vi "Analysis Vol. 3 CSV Read.vi"() -> ()   [LabVIEW 2014] (continued)
        n138 = Bundle(w213, w212) -> (w214:cluster{dbl, dbl})  [unwired: 1 in]
        n139 = Delete From Array(array=w183, index (row)=0 ("disabled index (col)")) -> (array with subset deleted=w233:dbl[][])  [unwired: 2 in, 1 out]
        n140 = property on="Choose Range:" class="Slide (strict)"("Scale.Maximum"=w213, "Scale.Minimum"=w212, "Value"=w214) -> ()  [unwired: 2 in, 2 out]
        n141 = property on="Range 2" class="Slide (strict)"("Scale.Maximum"=w213) -> ()  [unwired: 2 in, 2 out]
        n142 = property on="Range 3" class="Slide (strict)"("Scale.Maximum"=w213) -> ()  [unwired: 2 in, 2 out]
        n143 = property on="Range 4" class="Slide (strict)"("Scale.Maximum"=w213) -> ()  [unwired: 2 in, 2 out]
        n144 = Reshape Array("Well Names", w227) -> (w224:string[])
        n145 = Reshape Array("Concetrations", w227) -> (w228:dbl[])
        n146 = local read "96-well"() -> (w241:bool[][])
        n147 = Reshape Array(w241, w221) -> (w219:bool[])
        n148 = Decrement(x=w221) -> (x-1=w222:i32)
        n149 = Reverse 1D Array(array=w219) -> (reversed array=w220:bool[])
        n150 = for {
          shift-right: [w274] -> w236
          shift-left: w234 -> [w269]
          shift-right: [w272] -> w237
          shift-left: w233 -> [w273]
          shift-right: [w270] -> w217
          shift-left: w218 -> [w271]
          tunnel: w220 -> [w268] mode=indexing
          tunnel: w222 -> [w265]
          shift-right: [w263] -> w225
          shift-left: w224 -> [w264]
          shift-right: [w261] -> w229
          shift-left: w228 -> [w262]
          i -> [w267]
          n151 = Subtract(x=w265, y=w267) -> (x-y=w266:i32)
          n152 = case shown="False" w268 {
            tunnel: w269 -> [w284 w290]
            tunnel: [w285 w290] -> w274
            tunnel: w273 -> [w283 w289]
            tunnel: [w282 w289] -> w272
            tunnel: w271 -> [w281 w288]
            tunnel: [w280 w288] -> w270
            tunnel: w266 -> [w276 _]
            tunnel: w264 -> [w279 w287]
            tunnel: [w278 w287] -> w263
            tunnel: [w275 w286] -> w261
            tunnel: w262 -> [w277 w286]
            frame False {
              n153 = Delete From Array(array=w284, index (row)=w276) -> (array with subset deleted=w285:dbl[][])  [unwired: 2 in, 1 out]
              n154 = Delete From Array(array=w283, index (row)=w276) -> (array with subset deleted=w282:dbl[][])  [unwired: 2 in, 1 out]
              n155 = Delete From Array(array=w281, index (row)=w276) -> (array with subset deleted=w280:dbl[][])  [unwired: 2 in, 1 out]
              n156 = Delete From Array(array=w279, index=w276) -> (array with subset deleted=w278:string[])  [unwired: 1 in, 1 out]
              n157 = Delete From Array(array=w277, index=w276) -> (array with subset deleted=w275:dbl[])  [unwired: 1 in, 1 out]
            }
            frame True {
            }
          }
        }
        "Well Names" <- w225
        "Concetrations" <- w229
        "Dye 1/Melting" <- w236
        "Dye 2" <- w237
        "reference" <- w217
        n158 = for {
          tunnel: w216 -> [w260]
          tunnel: w236 -> [w259] mode=indexing
          tunnel: w237 -> [w258] mode=indexing
          tunnel: [w257] -> w238 mode=indexing
          tunnel: [w256] -> w239 mode=indexing
          tunnel: [w255] -> w240 mode=indexing
          n159 = Bundle(w260, w259) -> (w257:cluster{dbl[], dbl[]})  [unwired: 1 in]
          n160 = Bundle(w260, w258) -> (w256:cluster{dbl[], dbl[]})  [unwired: 1 in]
          n161 = Bundle(w260, w259) -> (w255:cluster{dbl[], dbl[]})  [unwired: 1 in]
        }
        "Dye 2: G1" <- w239
        "Dye 1: G1" <- w238
        "Melting G1" <- w240
        n162 = for {
          tunnel: w217 -> [w254] mode=indexing
          tunnel: [w253] -> w215 mode=indexing
          tunnel: w216 -> [w252]
          n163 = Bundle(w252, w254) -> (w253:cluster{dbl[], dbl[]})  [unwired: 1 in]
        }
        "REFERENCE G" <- w215
      }
      event "Range 2": Value Change {
        n164 = event-data() -> ()  [unwired: 1 in, 1 out]
        n165 = Unbundle("Range 2") -> (w294:dbl, w293:dbl)
        n166 = Max & Min(x=w294, y=w293) -> (max(x,y)=w292:dbl, min(x,y)=w291:dbl)
        n167 = property on="Dye1: G2" class="XYGraph (strict)"("XScale.Maximum"=w292, "XScale.Minimum"=w291) -> ()  [unwired: 2 in, 2 out]
      }
      event "Range 3": Value Change {
        n168 = event-data() -> ()  [unwired: 1 in, 1 out]
        n169 = Unbundle("Range 3") -> (w296:dbl, w297:dbl)
        n170 = Max & Min(x=w296, y=w297) -> (max(x,y)=w298:dbl, min(x,y)=w299:dbl)
        n171 = property on="Dye 5" class="XYGraph (strict)"("XScale.Maximum"=w298, "XScale.Minimum"=w299) -> ()  [unwired: 2 in, 2 out]
      }
      event "Range 4": Value Change {
        n172 = event-data() -> ()  [unwired: 1 in, 1 out]
        n173 = Unbundle("Range 4") -> (w301:dbl, w302:dbl)
        n174 = Max & Min(x=w301, y=w302) -> (max(x,y)=w304:dbl, min(x,y)=w305:dbl)
        n175 = property on="Dye1: G4" class="XYGraph (strict)"("XScale.Maximum"=w304, "XScale.Minimum"=w305) -> ()  [unwired: 2 in, 2 out]
      }
      event "Melting G1", "Melting G2", "Melting: G3": Cursor Move; "Intercalating/\nQuenching", "T[°C]", "conc [nM]": Value Change {
        w350 = 0.0019872041  # R
        w361 = 273.15
        # "lower T [°C]"
        # "points between\ncursors in G3"
        # "Jean-Louis Mergny and Laurent Lacroix. \nOligonucleotides. December 2003,\n13(6): 515-537. \ndoi:10.1089/154545703322860825."
        # "cursor pair green"
        # "cursor pair yellow"
        # "Fit baselines with cursors and make a bound fraction\nplot out of the meltcurve"
        # "stepsize"
        n176 = event-data() -> ()  [unwired: 1 in, 1 out]
        n177 = local read "Temp/Time\nranged"() -> (w324:dbl[])
        n178 = local read "Dye1/Melting ranged"() -> (w329:dbl[][])
        n179 = property on="Melting G1" class="XYGraph (strict)"("Active Cursor"=u32 0, "Active Cursor"=u32 1) -> ("Cursor.Cursor X"=w385:dbl, "Cursor.Cursor X"=w384:dbl)  [unwired: 2 in, 2 out]
        n180 = property on="Melting G3" class="XYGraph (strict)"("Active Cursor"=u32 1, "Active Cursor"=u32 0) -> ("Cursor.Cursor X"=w365:dbl, "Cursor.Cursor X"=w364:dbl)  [unwired: 2 in, 2 out]
        n181 = property on="Melting G1" class="XYGraph (strict)"("Active Cursor"=u32 2, "Active Cursor"=u32 3) -> ("Cursor.Cursor X"=w376:dbl, "Cursor.Cursor X"=w375:dbl)  [unwired: 2 in, 2 out]
        n182 = Index Array(array=w324, index=1) -> (element=w381:dbl)
        n183 = Index Array(array=w324, index=0) -> (element=w380:dbl)
        n184 = Subtract(x=w381, y=w380) -> ()  [unwired: 1 out]
        n185 = Reciprocal(x=w365) -> (1/x=w363:dbl)
        n186 = Reciprocal(x=w364) -> (1/x=w362:dbl)
        n187 = Max & Min(x=w385, y=w384) -> (max(x,y)=w336:dbl, min(x,y)=w335:dbl)
        n188 = Max & Min(x=w376, y=w375) -> (max(x,y)=w342:dbl, min(x,y)=w343:dbl)
        n189 = Subtract(x=w363, y=w361) -> (x-y=w359:dbl)
        n190 = Subtract(x=w362, y=w361) -> (x-y=w360:dbl)
        n191 = Max & Min(x=w359, y=w360) -> (max(x,y)=w325:dbl, min(x,y)=w316:dbl)
        "Upper T [°C]" <- w325
        "Lower T [°C]" <- w316
        n192 = Threshold 1D Array(2:w343, 3:w324) -> (0:w340:dbl)  [unwired: 1 in]
        n193 = Threshold 1D Array(2:w342, 3:w324) -> (0:w341:dbl)  [unwired: 1 in]
        n194 = Threshold 1D Array(2:w335, 3:w324) -> (0:w333:dbl)  [unwired: 1 in]
        n195 = Threshold 1D Array(2:w336, 3:w324) -> (0:w334:dbl)  [unwired: 1 in]
        n196 = Round Toward +Infinity(x=w341) -> (ceil(x): smallest int >= x=w338:dbl)
        n197 = Round Toward -Infinity(1:w340) -> (0:w337:dbl)
        n198 = Round Toward +Infinity(x=w334) -> (ceil(x): smallest int >= x=w332:dbl)
        n199 = Round Toward -Infinity(1:w333) -> (0:w331:dbl)
        n200 = Threshold 1D Array(2:w316, 3:w324) -> (0:w322:dbl)  [unwired: 1 in]
        n201 = Threshold 1D Array(2:w325, 3:w324) -> (0:w323:dbl)  [unwired: 1 in]
        n202 = Subtract(x=w338, y=w337) -> (x-y=w339:dbl)
        n203 = Subtract(x=w332, y=w331) -> (x-y=w327:dbl)
        n204 = Increment(x=w327) -> (x+1=w326:dbl)
        n205 = Round Toward +Infinity(x=w323) -> (ceil(x): smallest int >= x=w321:dbl)
        n206 = Round Toward -Infinity(1:w322) -> (0:w318:dbl)
        n207 = Increment(x=w339) -> (x+1=w328:dbl)
        n208 = property on="Melting G2" class="XYGraph (strict)"("Active Cursor"=u32 0, "Active Cursor"=u32 1) -> ("Cursor.Cursor X"=w371:dbl, "Cursor.Cursor Y"=w310:dbl, "Cursor.Cursor X"=w370:dbl, "Cursor.Cursor Y"=w309:dbl)  [unwired: 2 in, 2 out]
        n209 = Subtract(x=w321, y=w318) -> (x-y=w320:dbl)
        n210 = Increment(x=w320) -> (x+1=w319:dbl)
        n211 = Array Subset(array=w329, index (col)=w331, length (col)=w326) -> (w387:dbl[][])  [unwired: 2 in]
        "Baseline1" <- w387
        n212 = Array Subset(array=w324, index=w331, length=w326) -> (w386:dbl[])
        "Baseline1T" <- w386
        n213 = Array Subset(array=w329, index (col)=w337, length (col)=w328) -> (w374:dbl[][])  [unwired: 2 in]
        "Baseline2" <- w374
        n214 = Array Subset(array=w324, index=w337, length=w328) -> (w373:dbl[])
        "Baseline2T" <- w373
        n215 = Max & Min(x=w310, y=w309) -> (max(x,y)=→"Upper fraction":dbl, min(x,y)=→"Lower fraction":dbl)
        n216 = local read "Dye 1: G1"() -> (w379:cluster{"Y":dbl[], "Y":dbl[]}[])
        n217 = for {
          tunnel: w387 -> [w453] mode=indexing
          tunnel: w386 -> [w450]
          shift-right: [w452] -> w330
          shift-left: w379 -> [w407]
          tunnel: w329 -> [w437] mode=indexing
          tunnel: w374 -> [w449] mode=indexing
          tunnel: w373 -> [w447]
          tunnel: w324 -> [w398]
          tunnel: w343 -> [w441]
          tunnel: w335 -> [w440]
          tunnel: [w439] -> w372 mode=indexing
          tunnel: w371 -> [w435]
          tunnel: w370 -> [w434]
          tunnel: w316 -> [w394]
          tunnel: w319 -> [w423]
          tunnel: [w415] -> w367 mode=indexing
          tunnel: [w413] -> w352 mode=indexing
          tunnel: [w412] -> w353 mode=indexing
          tunnel: [w410] -> w358 mode=indexing
          tunnel: [w409] -> w357 mode=indexing
          tunnel: [w408] -> w356 mode=indexing
          tunnel: [w396] -> w317 mode=indexing
          w419 = 0.0019872041  # R
          w430 = 1e-09 ("x")
          # "lower T [°C]"
          # "ln(Ka) between cursors in G3"
          # "1/Temp between cursors in G3"
          # "Graph 3"
          # "fraction \nbound"
          # "index of lower T in G3"
          # "points between\ncursors in G3"
          # "Temp between cursors in G2"
          # "Fraction=(Higher Baseline - Signal)\n/(Higher Baseline - Lower Baseline)"
          # "green baseline"
          # "yellow baseline"
          # "which baseline is upper?"
          # "meltcurve"
          n218 = local read "Intercalating/\nQuenching"() -> (w436:bool)
          n219 = Max & Min(x=w435, y=w434) -> (max(x,y)=w391:dbl, min(x,y)=w390:dbl)
          n220 = call <vilib>:"Linear Fit.vi"("Y"=w453, "X"=w450) -> ("Best Linear Fit"=w451:dbl[], "slope"=w442:dbl, "intercept"=w443:dbl)  [unwired: 9 in, 2 out]
          n221 = call <vilib>:"Linear Fit.vi"("Y"=w449, "X"=w447) -> ("Best Linear Fit"=w448:dbl[], "slope"=w444:dbl, "intercept"=w445:dbl)  [unwired: 9 in, 2 out]
          n222 = for {
            tunnel: w443 -> [w473]
            tunnel: w442 -> [w476]
            tunnel: [w474] -> w401 mode=indexing
            tunnel: w398 -> [w472] mode=indexing
            n223 = Multiply(x=w476, y=w472) -> (x*y=w475:dbl)
            n224 = Add(x=w473, y=w475) -> (x+y=w474:dbl)
          }
          n225 = case shown="False" w436 {
            tunnel: [w454 w459] -> w400
            tunnel: w441 -> [w456 w458]
            tunnel: w440 -> [w455 w457]
            frame False {
              n226 = Greater?(x=w456, y=w455) -> (0:w454:bool)
            }
            frame True {
              n227 = Less?(x=w458, y=w457) -> (x < y?=w459:bool)
            }
          }
          n228 = for {
            tunnel: w445 -> [w477]
            tunnel: w444 -> [w479]
            tunnel: [w481] -> w438 mode=indexing
            tunnel: w398 -> [w480] mode=indexing
            # "stretch the fit over the \nwhole x-axis"
            n229 = Multiply(x=w480, y=w479) -> (x*y=w478:dbl)
            n230 = Add(x=w478, y=w477) -> (x+y=w481:dbl)
          }
          n231 = Bundle(w450, "Best Linear Fit"=w451) -> (w399:cluster{dbl[], "Best Linear Fit":dbl[]})  [unwired: 1 in]
          n232 = Bundle(w447, "Best Linear Fit"=w448) -> (w446:cluster{dbl[], "Best Linear Fit":dbl[]})  [unwired: 1 in]
          n233 = Threshold 1D Array(2:w390, 3:w398) -> (0:w405:dbl)  [unwired: 1 in]
          n234 = Threshold 1D Array(2:w391, 3:w398) -> (0:w406:dbl)  [unwired: 1 in]
          n235 = Insert Into Array(array=w407, new element #1=w446, new element #2=w399) -> (w452:cluster{"Y":dbl[], "Y":dbl[]}[])  [unwired: 1 in]
          n236 = Round Toward +Infinity(x=w406) -> (ceil(x): smallest int >= x=w404:dbl)
          n237 = Round Toward -Infinity(1:w405) -> (0:w403:dbl)
          n238 = Subtract(x=w404, y=w403) -> (x-y=w402:dbl)
          n239 = Increment(x=w402) -> (x+1=w397:dbl)
          n240 = Array Subset(array=w398, index=w403, length=w397) -> (w395:dbl[])
          n241 = case shown="False" w400 {
            tunnel: w437 -> [w462 w468]
            tunnel: w401 -> [w460 w467]
            tunnel: w438 -> [w461 w466]
            tunnel: [w463 w469] -> w410
            frame False {
              n242 = Subtract(x=w461, y=w460) -> (x-y=w464:dbl[])
              n243 = Subtract(x=w461, y=w462) -> (x-y=w465:dbl[])
              n244 = Divide(x=w465, y=w464) -> (x/y=w463:dbl[])
            }
            frame True {
              n245 = Subtract(x=w467, y=w468) -> (x-y=w471:dbl[])
              n246 = Subtract(x=w467, y=w466) -> (x-y=w470:dbl[])
              n247 = Divide(x=w471, y=w470) -> (x/y=w469:dbl[])
            }
          }
          n248 = Threshold 1D Array(2:w394, 3:w395) -> (0:w393:dbl)  [unwired: 1 in]
          n249 = Add(x=w395, y=273.15) -> (x+y=w433:dbl[])
          n250 = Reciprocal(x=w433) -> (1/x=w422:dbl[])
          "1/K" <- w422
          n251 = Round Toward -Infinity(1:w393) -> (0:w392:dbl)
          n252 = Array Subset(array=w410, index=w403, length=w397) -> (w411:dbl[])
          n253 = Bundle("Temp/Time\nranged"=w398, w410) -> (w439:cluster{"Temp/Time\nranged":dbl[], dbl[]})  [unwired: 1 in]
          n254 = Subtract(x=w411, y=1) -> (x-y=w431:dbl[])
          n255 = Compound Arithmetic op=MULTIPLY(w431, w430, "conc [nM]") -> (w428:dbl[])
          n256 = Compound Arithmetic op=MULTIPLY(w411, w430, "conc [nM]") -> (w425:dbl[])
          n257 = Square(x=w428) -> (x^2=w427:dbl[])
          n258 = Reciprocal(x=w427) -> (1/x=w426:dbl[])
          n259 = Multiply(x=w426, y=w425) -> (x*y=w424:dbl[])
          n260 = Natural Logarithm(1:w424) -> (0:w409:dbl[])
          n261 = Bundle(w422, w409) -> (w415:cluster{dbl[], dbl[]})  [unwired: 1 in]
          n262 = Array Subset(array=w409, index=w392, length=w423) -> (w417:dbl[])
          n263 = Array Subset(array=w422, index=w392, length=w423) -> (w416:dbl[])
          "ArrhFitT" <- w416
          n264 = call <vilib>:"Linear Fit.vi"("Y"=w417, "X"=w416) -> ("Best Linear Fit"=w408:dbl[], "slope"=w418:dbl, "intercept"=w421:dbl)  [unwired: 9 in, 2 out]
          n265 = Bundle(w416, "Best Linear Fit"=w408) -> (w396:cluster{dbl[], "Best Linear Fit":dbl[]})  [unwired: 1 in]
          n266 = Multiply(x=w419, y=w418) -> (x*y=w414:dbl)
          n267 = Multiply(x=w421, y=w419) -> (x*y=w412:dbl)
          n268 = Negate(x=w414) -> (-x=w413:dbl)
        }
        "Melting G2" <- w372
        "deltaH\n[kcal/mol]" <- w352
        "deltaS \n[kcal/K*mol]" <- w353
        "Bound Fraction" <- w358
        "ArrhLn" <- w357
        "ArrhFit" <- w356
        n269 = Insert Into Array(array=w367, new element=w317) -> (→"Melting: G3":cluster{dbl[], dbl[]}[])  [unwired: 1 in]
        n270 = local write "Melting G1"(w330) -> ()
        n271 = Add(x="T[°C]", y=273.15) -> (x+y=w307:dbl)
        n272 = Multiply(x=w353, y=w307) -> (x*y=w351:dbl[])
        n273 = Subtract(x=w352, y=w351) -> (x-y=w308:dbl[])
        "deltaG(T)\n[kcal/mol]" <- w308
        n274 = Multiply(x=w307, y=w350) -> (x*y=w306:dbl)
        n275 = Divide(x=w308, y=w306) -> (x/y=w349:dbl[])
        n276 = Exponential(1:w349) -> (0:w348:dbl[])
        n277 = Multiply(x=1000000000, y=w348) -> (x*y=w314:dbl[])
        "Kd\n[nM]" <- w314
        n278 = Multiply(x=w314, y="kon [1/(s*nM)]") -> (x*y=→"koff \n[1/s]":dbl[])
        n279 = Reciprocal(x=w314) -> (1/x=→"Ka\n[1/nM]":dbl[])
      }
      event "To Igor Meltcurve": Value Change {
        n280 = event-data() -> ()  [unwired: 1 in, 6 out]
        n281 = case shown="True" "Melting Curves" {
          frame False {
          }
          frame True {
            n282 = local read "Dye1/Melting ranged"() -> (w547:dbl[][])
            n283 = local read "Dye 1/Melting"() -> (w539:dbl[][])
            n284 = local read "Well Names"() -> (w540:string[])
            n285 = local read "Baseline2"() -> (w541:dbl[][])
            n286 = local read "Baseline1"() -> (w542:dbl[][])
            n287 = local read "Temp/Time\nranged"() -> (w548:dbl[])
            n288 = local read "Temp/Time"() -> (w537:dbl[])
            n289 = local read "Baseline1T"() -> (w543:dbl[])
            n290 = local read "Baseline2T"() -> (w544:dbl[])
            n291 = for {
              tunnel: w540 -> [w551] mode=indexing
              tunnel: w539 -> [w550] mode=indexing
              n292 = Concatenate Strings("Melt_raw_" ("string"), w551) -> (w553:string)
              n293 = call "1D_Data_to_Igor.vi"("Wave Name"=w553, "Data"=w550) -> ()  [unwired: 9 in, 1 out]
            }
            n294 = for {
              tunnel: w540 -> [w563] mode=indexing
              tunnel: w547 -> [w562] mode=indexing
              n295 = Concatenate Strings("Melt_cut_" ("string"), w563) -> (w565:string)
              n296 = call "1D_Data_to_Igor.vi"("Wave Name"=w565, "Data"=w562) -> ()  [unwired: 9 in, 1 out]
            }
            n297 = for {
              tunnel: w540 -> [w559] mode=indexing
              tunnel: w541 -> [w558] mode=indexing
              n298 = Concatenate Strings("Melt_BL2_" ("string"), w559) -> (w561:string)
              n299 = call "1D_Data_to_Igor.vi"("Wave Name"=w561, "Data"=w558) -> ()  [unwired: 9 in, 1 out]
            }
            n300 = for {
              tunnel: w540 -> [w555] mode=indexing
              tunnel: w542 -> [w554] mode=indexing
              n301 = Concatenate Strings("Melt_BL1_" ("string"), w555) -> (w557:string)
              n302 = call "1D_Data_to_Igor.vi"("Wave Name"=w557, "Data"=w554) -> ()  [unwired: 9 in, 1 out]
            }
            n303 = call "1D_Data_to_Igor.vi"("Wave Name"="Melt_cut_Temperature" ("string"), "Data"=w548) -> ()  [unwired: 9 in, 1 out]
            n304 = call "1D_Data_to_Igor.vi"("Wave Name"="Melt_TemperatureBL1" ("string"), "Data"=w543) -> ()  [unwired: 9 in, 1 out]
            n305 = call "1D_Data_to_Igor.vi"("Wave Name"="Melt_TemperatureBL2" ("string"), "Data"=w544) -> ()  [unwired: 9 in, 1 out]
            n306 = call "1D_Data_to_Igor.vi"("Wave Name"="Melt_raw_Temperature" ("string"), "Data"=w537) -> ()  [unwired: 9 in, 1 out]
          }
        }
        n307 = case shown="True" "Bound Fraction" {
          frame False {
          }
          frame True {
            n308 = local read "Bound Fraction"() -> (w530:dbl[][])
            n309 = local read "Temp/Time\nranged"() -> (w529:dbl[])
            n310 = local read "Well Names"() -> (w531:string[])
            n311 = for {
              tunnel: w531 -> [w534] mode=indexing
              tunnel: w530 -> [w533] mode=indexing
              n312 = Concatenate Strings("Fraction_" ("string"), w534) -> (w536:string)
              n313 = call "1D_Data_to_Igor.vi"("Wave Name"=w536, "Data"=w533) -> ()  [unwired: 9 in, 1 out]
            }
            n314 = call "1D_Data_to_Igor.vi"("Wave Name"="Fraction_Temperature" ("string"), "Data"=w529) -> ()  [unwired: 9 in, 1 out]
          }
        }
        n315 = case shown="True" "Arrhenius Plot" {
          frame False {
          }
          frame True {
            n316 = local read "Well Names"() -> (w520:string[])
            n317 = local read "ArrhFit"() -> (w515:dbl[][])
            n318 = local read "ArrhLn"() -> (w518:dbl[][])
            n319 = for {
              tunnel: w520 -> [w522] mode=indexing
              tunnel: w518 -> [w526] mode=indexing
              tunnel: w515 -> [w524] mode=indexing
              n320 = Concatenate Strings("ArrhFit_" ("string"), w522) -> (w525:string)
              n321 = Concatenate Strings("Arrh_" ("string"), w522) -> (w528:string)
              n322 = call "1D_Data_to_Igor.vi"("Wave Name"=w525, "Data"=w524) -> ()  [unwired: 9 in, 1 out]
              n323 = call "1D_Data_to_Igor.vi"("Wave Name"=w528, "Data"=w526) -> ()  [unwired: 9 in, 1 out]
            }
            n324 = local read "ArrhFitT"() -> (w516:dbl[])
            n325 = local read "1/K"() -> (w519:dbl[])
            n326 = call "1D_Data_to_Igor.vi"("Wave Name"="Arrh_invT" ("string"), "Data"=w519) -> ()  [unwired: 9 in, 1 out]
            n327 = call "1D_Data_to_Igor.vi"("Wave Name"="ArrhFit_invT" ("string"), "Data"=w516) -> ()  [unwired: 9 in, 1 out]
          }
        }
        n328 = case shown="True" "Energies & Kd, Ka" {
          frame False {
          }
          frame True {
            w490 = "_" ("string")
            n329 = local read "kon [1/(s*nM)]"() -> (w488:dbl)
            n330 = local read "conc [nM]"() -> (w497:dbl)
            n331 = local read "deltaS \n[kcal/K*mol]"() -> (w514:dbl[])
            n332 = local read "T[°C]"() -> (w507:dbl)
            n333 = local read "deltaH\n[kcal/mol]"() -> (w510:dbl[])
            n334 = local read "Well Names"() -> (w500:string[])
            n335 = Number To Decimal String(number=w507) -> (decimal integer string=w499:string)  [unwired: 1 in]
            n336 = Number To Decimal String(number=w497) -> (decimal integer string=w491:string)  [unwired: 1 in]
            n337 = Number To Fractional String(number=w488, width (-)=5, precision (6)=4) -> (F-format string=w489:string)  [unwired: 1 in]
            n338 = call "1D_Strings_to_Igor_with_Prefix.vi"("Wave Name"="Samples" ("string"), "Data"=w500) -> ()  [unwired: 9 in, 1 out]
            n339 = call "1D_Data_to_Igor.vi"("Wave Name"="deltaS_kcal_K_mol" ("string"), "Data"=w514) -> ()  [unwired: 9 in, 1 out]
            n340 = call "1D_Data_to_Igor.vi"("Wave Name"="deltaH_kcal_mol" ("string"), "Data"=w510) -> ()  [unwired: 9 in, 1 out]
            n341 = local read "deltaG(T)\n[kcal/mol]"() -> (w511:dbl[])
            n342 = Concatenate Strings("deltaG_kcal_mol_" ("string"), w499) -> (w502:string)
            n343 = Concatenate Strings("koff_" ("string"), w499, w490, w491, w490, w489) -> (w493:string)
            n344 = local read "koff \n[1/s]"() -> (w498:dbl[])
            n345 = call "1D_Data_to_Igor.vi"("Wave Name"=w502, "Data"=w511) -> ()  [unwired: 9 in, 1 out]
            n346 = call "1D_Data_to_Igor.vi"("Wave Name"=w493, "Data"=w498) -> ()  [unwired: 9 in, 1 out]
            n347 = Concatenate Strings("Kd_nM_" ("string"), w499, "_" ("string"), w491) -> (w495:string)
            n348 = Concatenate Strings("Ka_nM_" ("string"), w499, "_" ("string"), w491) -> (w505:string)
            n349 = local read "Kd\n[nM]"() -> (w508:dbl[])
            n350 = local read "Ka\n[1/nM]"() -> (w509:dbl[])
            n351 = call "1D_Data_to_Igor.vi"("Wave Name"=w495, "Data"=w508) -> ()  [unwired: 9 in, 1 out]
            n352 = call "1D_Data_to_Igor.vi"("Wave Name"=w505, "Data"=w509) -> ()  [unwired: 9 in, 1 out]
          }
        }
      }
      event "Row": Value Change {
        n353 = event-data() -> ("NewVal"=w581:bool[], "OldVal"=w580:bool[])  [unwired: 1 in]
        n354 = Boolean To (0,1)(Boolean=w581) -> (0, 1=w579:i16[])
        n355 = Boolean To (0,1)(Boolean=w580) -> (0, 1=w578:i16[])
        n356 = Subtract(x=w579, y=w578) -> (x-y=w577:i16[])
        n357 = Absolute Value(x=w577) -> (abs(x)=w576:i16[])
        n358 = Array Max & Min(array=w576) -> (max index (indices)=w569:i32)  [unwired: 3 out]
        n359 = Index Array(array="96-well", index (row)=w569) -> (element=w570:bool[])  [unwired: 1 in]
        n360 = Boolean To (0,1)(Boolean=w570) -> (0, 1=w571:i16[])
        n361 = Multiply Array Elements(1:w571) -> (0:w572:i16)
        n362 = Equal To 0?(x=w572) -> (x = 0?=w573:bool)
        n363 = Select(t=bool[] [TRUE, TRUE, TRUE, TRUE, TRUE, TRUE, TRUE, TRUE, TRUE, TRUE, TRUE, TRUE] ("new element/subarray"), s=w573, f=bool[] [FALSE, FALSE, FALSE, FALSE, FALSE, FALSE, FALSE, FALSE, FALSE, FALSE, FALSE, FALSE] ("new element/subarray")) -> (s? t:f=w574:bool[])
        n364 = Replace Array Subset(array="96-well", new element=w574, index (row)=w569) -> (w575:bool[][])  [unwired: 1 in]
        n365 = local write "96-well"(w575) -> ()
      }
      event "All": Value Change {
        n366 = event-data() -> ()  [unwired: 1 in, 1 out]
        n367 = local read "96-well"() -> (w582:bool[][])
        n368 = Boolean To (0,1)(Boolean=w582) -> (0, 1=w588:i16[][])
        n369 = Multiply Array Elements(1:w588) -> (0:w586:i16)
        n370 = Equal To 0?(x=w586) -> (x = 0?=w585:bool)
        n371 = Select(t=bool[][] [[TRUE, TRUE, TRUE, TRUE, TRUE, TRUE, TRUE, TRUE, TRUE, TRUE, TRUE, TRUE], [TRUE, TRUE, TRUE, TRUE, TRUE, TRUE, TRUE, TRUE, TRUE, TRUE, TRUE, TRUE], [TRUE, TRUE, TRUE, TRUE, TRUE, TRUE, TRUE, TRUE, TRUE, TRUE, TRUE, TRUE], [TRUE, TRUE, TRUE, TRUE, TRUE, TRUE, TRUE, TRUE, TRUE, TRUE, TRUE, TRUE], [TRUE, TRUE, TRUE, TRUE, TRUE, TRUE, TRUE, TRUE, TRUE, TRUE, TRUE, TRUE], [TRUE, TRUE, TRUE, TRUE, TRUE, TRUE, TRUE, TRUE, TRUE, TRUE, TRUE, TRUE], [TRUE, TRUE, TRUE, TRUE, TRUE, TRUE, TRUE, TRUE, TRUE, TRUE, TRUE, TRUE], [TRUE, TRUE, TRUE, TRUE, TRUE, TRUE, TRUE, TRUE, TRUE, TRUE, TRUE, TRUE]] ("96-well 2"), s=w585, f=bool[][] [[FALSE, FALSE, FALSE, FALSE, FALSE, FALSE, FALSE, FALSE, FALSE, FALSE, FALSE, FALSE], [FALSE, FALSE, FALSE, FALSE, FALSE, FALSE, FALSE, FALSE, FALSE, FALSE, FALSE, FALSE], [FALSE, FALSE, FALSE, FALSE, FALSE, FALSE, FALSE, FALSE, FALSE, FALSE, FALSE, FALSE], [FALSE, FALSE, FALSE, FALSE, FALSE, FALSE, FALSE, FALSE, FALSE, FALSE, FALSE, FALSE], [FALSE, FALSE, FALSE, FALSE, FALSE, FALSE, FALSE, FALSE, FALSE, FALSE, FALSE, FALSE], [FALSE, FALSE, FALSE, FALSE, FALSE, FALSE, FALSE, FALSE, FALSE, FALSE, FALSE, FALSE], [FALSE, FALSE, FALSE, FALSE, FALSE, FALSE, FALSE, FALSE, FALSE, FALSE, FALSE, FALSE], [FALSE, FALSE, FALSE, FALSE, FALSE, FALSE, FALSE, FALSE, FALSE, FALSE, FALSE, FALSE]] ("96-well 2")) -> (s? t:f=w587:bool[][])
        n372 = local write "96-well"(w587) -> ()
      }
      event "Line": Value Change {
        n373 = event-data() -> ("NewVal"=w604:bool[], "OldVal"=w603:bool[])  [unwired: 1 in]
        n374 = Boolean To (0,1)(Boolean=w604) -> (0, 1=w602:i16[])
        n375 = Boolean To (0,1)(Boolean=w603) -> (0, 1=w601:i16[])
        n376 = Subtract(x=w602, y=w601) -> (x-y=w600:i16[])
        n377 = Absolute Value(x=w600) -> (abs(x)=w599:i16[])
        n378 = local read "96-well"() -> (w589:bool[][])
        n379 = Array Max & Min(array=w599) -> (max index (indices)=w592:i32)  [unwired: 3 out]
        n380 = Index Array(array=w589, index (col)=w592) -> (element=w593:bool[])  [unwired: 1 in]
        n381 = Boolean To (0,1)(Boolean=w593) -> (0, 1=w594:i16[])
        n382 = Multiply Array Elements(1:w594) -> (0:w595:i16)
        n383 = Equal To 0?(x=w595) -> (x = 0?=w596:bool)
        n384 = Select(t=bool[] [TRUE, TRUE, TRUE, TRUE, TRUE, TRUE, TRUE, TRUE] ("Row 2"), s=w596, f=bool[] [FALSE, FALSE, FALSE, FALSE, FALSE, FALSE, FALSE, FALSE] ("Row 3")) -> (s? t:f=w597:bool[])
        n385 = Replace Array Subset(array=w589, new element=w597, index (col)=w592) -> (w598:bool[][])  [unwired: 1 in]
        n386 = local write "96-well"(w598) -> ()
      }
      event "96-well": Value Change {
        n387 = event-data() -> ()  [unwired: 1 in, 2 out]
        n388 = local read "Reference \non/off"() -> (w605:bool)
        n389 = property on="Reference \non/off" class="Bool (strict)"("Val(Sgnl)"=w605) -> ()  [unwired: 2 in, 2 out]
        n390 = local read "Load Dye 2"() -> (w606:path)
        n391 = property on="Load Dye 2" class="Path"("Val(Sgnl)"=w606) -> ()  [unwired: 2 in, 2 out]
      }
      event "Dye 1: G1": Cursor Move; "Update Dye1: G2": Value Change {
        # "Dye1array"
        n392 = event-data() -> ()  [unwired: 1 in, 1 out]
        n393 = local read "Dye1/Melting ranged"() -> (w607:dbl[][])
        n394 = case shown="True" "I - I0" {
          tunnel: w607 -> [w645 w647]
          tunnel: [w645 w646] -> w617
          frame False {
          }
          frame True {
            # "Subtrac I0"
            n395 = for {
              tunnel: w647 -> [w649] mode=indexing
              tunnel: [w648] -> w646 mode=indexing
              n396 = Index Array(array=w649, index=0) -> (element=w650:dbl)
              n397 = Subtract(x=w649, y=w650) -> (x-y=w648:dbl[])
            }
          }
        }
        n398 = local read "Temp/Time\nranged"() -> (w608:dbl[])
        n399 = case shown="True" "Baseline Correction" {
          tunnel: w617 -> [w656 w688]
          tunnel: w608 -> [w658 w681]
          tunnel: "Concentrations" -> [_ w685]
          tunnel: "Invert" -> [w655 w683]
          tunnel: [w656 w680] -> w615
          tunnel: [w657 w682] -> w614
          tunnel: "Normalize" -> [w653 w678]
          frame False {
            n400 = case shown="False" w655 {
              tunnel: [w667 w674] -> w654
              tunnel: w656 -> [w668 w674]
              frame True {
                n401 = for {
                  tunnel: w668 -> [w670] mode=indexing
                  tunnel: [w669] -> w667 mode=indexing
                  n402 = Array Max & Min(array=w670) -> (max value=w671:dbl)  [unwired: 3 out]
                  n403 = Multiply(x=w670, y=-1.0) -> (x*y=w672:dbl[])
                  n404 = Add(x=w672, y=w671) -> (x+y=w669:dbl[])
                }
              }
              frame False {
              }
            }
            n405 = case shown="True" w653 {
              tunnel: [w659 w660] -> w652
              tunnel: w654 -> [w659 w661]
              frame False {
              }
              frame True {
                n406 = for {
                  tunnel: w661 -> [w665] mode=indexing
                  tunnel: [w662] -> w660 mode=indexing
                  n407 = Array Max & Min(array=w665) -> (min value=w666:dbl)  [unwired: 3 out]
                  n408 = Subtract(x=w665, y=w666) -> (x-y=w663:dbl[])
                  n409 = Array Max & Min(array=w663) -> (max value=w664:dbl)  [unwired: 3 out]
                  n410 = Divide(x=w663, y=w664) -> (x/y=w662:dbl[])
                }
              }
            }
            n411 = local write "Dye1withBaselineCorrection"(w652) -> ()
            n412 = for {
              tunnel: [w677] -> w657 mode=indexing
              tunnel: w658 -> [w676]
              tunnel: w652 -> [w675] mode=indexing
              # "Create Plots"
              n413 = Bundle("Temp/Time\nranged"=w676, "Dye1/Melting ranged"=w675) -> (w677:T4)  [unwired: 1 in]
            }
            n414 = local write "Dye1: G2"(w657) -> ()
          }
          frame True {
            # "I-I0"
            n415 = property on="Dye 1: G1" class="XYGraph (strict)"("Active Cursor"=u32 0, "Active Cursor"=u32 1) -> ("Cursor.Cursor X"=w699:dbl, "Cursor.Cursor X"=w700:dbl)  [unwired: 2 in, 2 out]
            n416 = Array Size(array=w688) -> (size(s)=w691:i32[])
            n417 = Index Array(array=w691, index=1) -> (element=w689:i32)
            n418 = Max & Min(x=w699, y=w700) -> (max(x,y)=w695:dbl, min(x,y)=w692:dbl)
            n419 = Subtract(x=w695, y=w692) -> (x-y=w693:dbl)
            n420 = Array Subset(array=w688, index (col)=w692, length (col)=w693) -> (w694:dbl[][])  [unwired: 2 in]
            n421 = Array Subset(array=w681, index=w692, length=w693) -> (w696:dbl[])
            n422 = for {
              tunnel: w694 -> [w752] mode=indexing
              tunnel: w696 -> [w751]
              tunnel: w689 -> [w750]
              tunnel: [w745] -> w687 mode=indexing
              n423 = call <vilib>:"Linear Fit.vi"("Y"=w752, "X"=w751) -> ("slope"=w746:dbl, "intercept"=w747:dbl)  [unwired: 9 in, 3 out]
              n424 = Initialize Array(w747, w750) -> (w749:dbl[])
              n425 = Decrement(x=w750) -> (x-1=w748:i32)
              n426 = for {
                N: w748 -> [_]
                shift-right: [w758] -> w745
                shift-left: w749 -> [w759]
                tunnel: w747 -> [w757]
                tunnel: w746 -> [w755]
                i -> [w760]
                n427 = Increment(x=w760) -> (x+1=w756:i32)
                n428 = Multiply(x=w755, y=w756) -> (x*y=w754:dbl)
                n429 = Add(x=w757, y=w754) -> (x+y=w753:dbl)
                n430 = Replace Array Subset(array=w759, new element=w753, index=w756) -> (w758:dbl[])
              }
            }
            n431 = local read "Concetrations"() -> (w684:dbl[])
            n432 = Divide(x=w688, y=w687) -> (x/y=w686:dbl[][])
            n433 = case shown="False" w685 {
              tunnel: [w709 w729] -> w679
              tunnel: w686 -> [w711 w731]
              tunnel: w684 -> [w712 w732]
              tunnel: w683 -> [w710 w730]
              frame True {
                n434 = for {
                  tunnel: w712 -> [w722] mode=indexing
                  tunnel: w711 -> [w721] mode=indexing
                  tunnel: w710 -> [w714]
                  tunnel: [w713] -> w709 mode=indexing
                  n435 = Array Max & Min(array=w721) -> (max value=w720:dbl, min value=w719:dbl)  [unwired: 2 out]
                  n436 = Subtract(x=w721, y=w719) -> (x-y=w717:dbl[])
                  n437 = Subtract(x=w720, y=w719) -> (x-y=w716:dbl)
                  n438 = Divide(x=w717, y=w716) -> (x/y=w718:dbl[])
                  n439 = Multiply(x=w718, y=w722) -> (x*y=w715:dbl[])
                  n440 = case shown="True" w714 {
                    tunnel: w715 -> [w723 w727]
                    tunnel: [w723 w724] -> w713
                    frame False {
                    }
                    frame True {
                      n441 = Array Max & Min(array=w727) -> (max value=w725:dbl)  [unwired: 3 out]
                      n442 = Multiply(x=w727, y=-1.0) -> (x*y=w726:dbl[])
                      n443 = Add(x=w726, y=w725) -> (x+y=w724:dbl[])
                    }
                  }
                }
              }
              frame False {
                n444 = for {
                  tunnel: w732 -> [_] mode=indexing
                  tunnel: w731 -> [w734] mode=indexing
                  tunnel: w730 -> [w733]
                  tunnel: [w735] -> w729 mode=indexing
                  n445 = case shown="False" w733 {
                    tunnel: w734 -> [w736 w740]
                    tunnel: [w736 w737] -> w735
                    frame False {
                    }
                    frame True {
                      n446 = Array Max & Min(array=w740) -> (max value=w738:dbl)  [unwired: 3 out]
                      n447 = Multiply(x=w740, y=-1.0) -> (x*y=w739:dbl[])
                      n448 = Add(x=w739, y=w738) -> (x+y=w737:dbl[])
                    }
                  }
                }
              }
            }
            n449 = case shown="True" w678 {
              tunnel: [w701 w702] -> w680
              tunnel: w679 -> [w701 w703]
              frame False {
              }
              frame True {
                n450 = for {
                  tunnel: w703 -> [w707] mode=indexing
                  tunnel: [w704] -> w702 mode=indexing
                  n451 = Array Max & Min(array=w707) -> (min value=w708:dbl)  [unwired: 3 out]
                  n452 = Subtract(x=w707, y=w708) -> (x-y=w705:dbl[])
                  n453 = Array Max & Min(array=w705) -> (max value=w706:dbl)  [unwired: 3 out]
                  n454 = Divide(x=w705, y=w706) -> (x/y=w704:dbl[])
                }
              }
            }
            "Dye1withBaselineCorrection" <- w680
            n455 = for {
              tunnel: [w744] -> w682 mode=indexing
              tunnel: w680 -> [w743] mode=indexing
              tunnel: w681 -> [w742]
              # "Create Plots"
              n456 = Bundle("Temp/Time\nranged"=w742, w743) -> (w744:cluster{"Temp/Time\nranged":dbl[], dbl[]})  [unwired: 1 in]
            }
            "Dye1: G2" <- w682
          }
        }
        n457 = case shown="True" w616 {
          tunnel: w608 -> [w624 _]
          tunnel: w615 -> [w619 _]
          tunnel: w614 -> [_ w644]
          frame True {
            w623 = cluster{"Y":dbl[], "Y":dbl[]}[] []  # Dye 3
            n458 = property on="Dye1: G2" class="XYGraph (strict)"("Active Cursor"=u32 0, "Active Cursor"=u32 1) -> ("Cursor.Cursor X"=w629:dbl, "Cursor.Cursor X"=w628:dbl)  [unwired: 2 in, 2 out]
            n459 = Max & Min(x=w629, y=w628) -> (max(x,y)=w631:dbl, min(x,y)=w630:dbl)
            n460 = Subtract(x=w631, y=w630) -> (x-y=w627:dbl)
            n461 = Array Subset(array=w619, index (col)=w630, length (col)=w627) -> (w625:dbl[][])  [unwired: 2 in]
            n462 = Array Subset(array=w624, index=w630, length=w627) -> (w626:dbl[])
            n463 = for {
              tunnel: w625 -> [w643] mode=indexing
              tunnel: w626 -> [w635]
              shift-right: [w641] -> w620
              shift-left: w623 -> [w640]
              tunnel: w624 -> [w638]
              tunnel: w619 -> [w637] mode=indexing
              tunnel: [w636] -> w622 mode=indexing
              tunnel: [w635] -> w621
              tunnel: [w634] -> w618 mode=indexing
              n464 = call <vilib>:"Linear Fit.vi"("Y"=w643, "X"=w635) -> ("Best Linear Fit"=w636:dbl[], "slope"=w634:dbl)  [unwired: 9 in, 3 out]
              n465 = Bundle("Temp/Time\nranged"=w638, "Dye1/Melting ranged"=w637) -> (w639:T4)  [unwired: 1 in]
              n466 = Bundle(w635, "Best Linear Fit"=w636) -> (w642:cluster{dbl[], "Best Linear Fit":dbl[]})  [unwired: 1 in]
              n467 = Insert Into Array(array=w640, new element #1=w642, new element #2=w639) -> (w641:cluster{"Y":dbl[], "Y":dbl[]}[])  [unwired: 1 in]
            }
            "FitDye1" <- w622
            "FitTimeDye1" <- w621
            "FitDye1Slopes" <- w618
            n468 = local write "Dye1: G2"(w620) -> ()
          }
          frame False {
            n469 = local write "Dye1: G2"(w644) -> ()
          }
        }
      }
      event "Update Dye1: G4": Value Change {
        n470 = event-data() -> ()  [unwired: 1 in, 6 out]
        n471 = local read "Dye1withBaselineCorrection"() -> (w763:dbl[][])
        n472 = local read "FitDye1"() -> (w764:dbl[][])
        n473 = for {
          tunnel: w764 -> [w773] mode=indexing
          tunnel: w763 -> [w778] mode=indexing
          tunnel: [w768] -> w762 mode=indexing
          n474 = Array Max & Min(array=w778) -> (max value=w769:dbl)  [unwired: 3 out]
          n475 = Add Array Elements(numeric array=w773) -> (sum=w774:dbl)
          n476 = Array Size(array=w773) -> (size(s)=w772:i32)
          n477 = Divide(x=w774, y=w772) -> (x/y=w770:dbl)
          n478 = Subtract(x=w778, y=w769) -> (x-y=w776:dbl[])
          n479 = Subtract(x=w770, y=w769) -> (x-y=w775:dbl)
          n480 = Divide(x=w776, y=w775) -> (x/y=w777:dbl[])
          n481 = Multiply(x=w777, y="Upper saturation conc (plateau)") -> (x*y=w766:dbl[])
          n482 = Add(x="Lower treshold conc", y=w766) -> (x+y=w768:dbl[])
        }
        n483 = local read "Temp/Time\nranged"() -> (w761:dbl[])
        n484 = for {
          tunnel: [w781] -> w765 mode=indexing
          tunnel: w762 -> [w780] mode=indexing
          tunnel: w761 -> [w779]
          # "Create Plots"
          n485 = Bundle("Temp/Time\nranged"=w779, w780) -> (w781:cluster{"Temp/Time\nranged":dbl[], dbl[]})  [unwired: 1 in]
        }
        "Dye1: G4" <- w765
      }
      event "Update Dye1: G3": Value Change {
        n486 = event-data() -> ()  [unwired: 1 in, 6 out]
        n487 = local read "Concetrations"() -> (w782:dbl[])
        "ConcentrationDye1" <- w782
        n488 = local read "FitDye1Slopes"() -> (w789:dbl[])
        n489 = Negate(x=w789) -> (-x=w788:dbl[])
        n490 = Select(t=w788, s="invert MM", f=w789) -> (s? t:f=w783:dbl[])
        "SlopesDye1" <- w783
        n491 = Bundle("Concetrations"=w782, "FitDye1Slopes"=w783) -> (w784:T5)  [unwired: 1 in]
        n492 = case shown="True" "Michaelis Menten Fit" {
          tunnel: w783 -> [_ w799]
          tunnel: [w791 w797] -> w785
          tunnel: w784 -> [w790 w793]
          tunnel: w782 -> [_ w795]
          frame False {
            n493 = Build Array "Build Array"(w790) -> (w791:T1)
          }
          frame True {
            n494 = call-poly <vilib>:"Nonlinear Curve Fit.vi"("Y"=w799, "initial parameters"="initial parameters", "X"=w795, "model description"=T3 {"model"="a1*x/(a2+x)", "Parameters"=["a1", "a2"], "x"="x"}) -> ("best nonlinear fit"=w796:dbl[], "best fit parameters"=→"best fit parameters 1":dbl[])  [unwired: 7 in, 3 out]
            "best nonlinear fit Dye1" <- w796
            n495 = Bundle("Concetrations"=w795, "best nonlinear fit"=w796) -> (w794:T6)  [unwired: 1 in]
            n496 = Build Array "Build Array"(w793, w794) -> (w797:T2)
          }
        }
        "Dye1: G3" <- w785
      }
      event "Update Dye2: G3": Value Change {
        n497 = event-data() -> ()  [unwired: 1 in, 6 out]
        n498 = local read "FitDye2Slopes"() -> (w803:dbl[])
        n499 = Negate(x=w803) -> (-x=w808:dbl[])
        n500 = local read "Concetrations"() -> (w801:dbl[])
        "ConcentrationDye2" <- w801
        n501 = Select(t=w808, s="invert MM 2", f=w803) -> (s? t:f=w805:dbl[])
        "SlopesDye2" <- w805
        n502 = Bundle("Concetrations"=w801, "FitDye2Slopes"=w805) -> (w806:T7)  [unwired: 1 in]
        n503 = case shown="True" "Michaelis Menten Fit 2" {
          tunnel: w805 -> [_ w818]
          tunnel: [w810 w816] -> w804
          tunnel: w806 -> [w809 w814]
          tunnel: w801 -> [_ w812]
          frame False {
            n504 = Build Array "Build Array"(w809) -> (w810:T8)
          }
          frame True {
            n505 = call-poly <vilib>:"Nonlinear Curve Fit.vi"("Y"=w818, "initial parameters"="initial parameters 2", "X"=w812, "model description"=T3 {"model"="a1*x/(a2+x)", "Parameters"=["a1", "a2"], "x"="x"}) -> ("best nonlinear fit"=w811:dbl[], "best fit parameters"=→"best fit parameters 2":dbl[])  [unwired: 7 in, 3 out]
            "best nonlinear fit Dye2" <- w811
            n506 = Bundle("Concetrations"=w812, "best nonlinear fit"=w811) -> (w815:T6)  [unwired: 1 in]
            n507 = Build Array "Build Array"(w814, w815) -> (w816:T2)
          }
        }
        "Dye2: G3" <- w804
      }
      event "Dye 2: G1": Cursor Move; "Update Dye2: G2": Value Change {
        n508 = event-data() -> ()  [unwired: 1 in, 1 out]
        n509 = local read "Temp/Time\nranged"() -> (w820:dbl[])
        n510 = local read "Dye2 ranged"() -> (w821:dbl[][])
        n511 = case shown="True" "I - I0" {
          tunnel: w821 -> [w859 w861]
          tunnel: [w859 w860] -> w831
          frame False {
          }
          frame True {
            n512 = for {
              tunnel: w861 -> [w863] mode=indexing
              tunnel: [w862] -> w860 mode=indexing
              n513 = Index Array(array=w863, index=0) -> (element=w864:dbl)
              n514 = Subtract(x=w863, y=w864) -> (x-y=w862:dbl[])
            }
          }
        }
        n515 = local read "Invert"() -> (w823:bool)
        n516 = case shown="True" "Baseline Correction" {
          tunnel: w831 -> [w868 w893]
          tunnel: w820 -> [w870 w891]
          tunnel: "Concentrations" -> [_ w889]
          tunnel: "Invert" -> [_ w887]
          tunnel: [w868 w883] -> w830
          tunnel: [w869 w886] -> w829
          tunnel: w823 -> [_ w885]
          tunnel: "Normalize" -> [w867 w882]
          frame False {
            n517 = case shown="True" w867 {
              tunnel: [w871 w873] -> w866
              tunnel: w868 -> [w871 w872]
              frame False {
              }
              frame True {
                n518 = for {
                  tunnel: w872 -> [w877] mode=indexing
                  tunnel: [w874] -> w873 mode=indexing
                  n519 = Array Max & Min(array=w877) -> (min value=w878:dbl)  [unwired: 3 out]
                  n520 = Subtract(x=w877, y=w878) -> (x-y=w875:dbl[])
                  n521 = Array Max & Min(array=w875) -> (max value=w876:dbl)  [unwired: 3 out]
                  n522 = Divide(x=w875, y=w876) -> (x/y=w874:dbl[])
                }
              }
            }
            n523 = local write "Dye2withBaselineCorrectio"(w866) -> ()
            n524 = for {
              tunnel: [w881] -> w869 mode=indexing
              tunnel: w870 -> [w880]
              tunnel: w866 -> [w879] mode=indexing
              # "Create Plots"
              n525 = Bundle("Temp/Time\nranged"=w880, "Dye2 ranged"=w879) -> (w881:T9)  [unwired: 1 in]
            }
            n526 = local write "Dye 5"(w869) -> ()
          }
          frame True {
            n527 = property on="Dye 2: G1" class="XYGraph (strict)"("Active Cursor"=u32 0, "Active Cursor"=u32 1) -> ("Cursor.Cursor X"=w904:dbl, "Cursor.Cursor X"=w905:dbl)  [unwired: 2 in, 2 out]
            n528 = Array Size(array=w893) -> (size(s)=w896:i32[])
            n529 = Index Array(array=w896, index=1) -> (element=w894:i32)
            n530 = Max & Min(x=w904, y=w905) -> (max(x,y)=w900:dbl, min(x,y)=w897:dbl)
            n531 = Subtract(x=w900, y=w897) -> (x-y=w898:dbl)
            n532 = Array Subset(array=w893, index (col)=w897, length (col)=w898) -> (w899:dbl[][])  [unwired: 2 in]
            n533 = Array Subset(array=w891, index=w897, length=w898) -> (w901:dbl[])
            n534 = for {
              tunnel: w899 -> [w956] mode=indexing
              tunnel: w901 -> [w955]
              tunnel: w894 -> [w954]
              tunnel: [w949] -> w892 mode=indexing
              n535 = call <vilib>:"Linear Fit.vi"("Y"=w956, "X"=w955) -> ("slope"=w950:dbl, "intercept"=w951:dbl)  [unwired: 9 in, 3 out]
              n536 = Initialize Array(w951, w954) -> (w953:dbl[])
              n537 = Decrement(x=w954) -> (x-1=w952:i32)
              n538 = for {
                N: w952 -> [_]
                shift-right: [w962] -> w949
                shift-left: w953 -> [w963]
                tunnel: w951 -> [w961]
                tunnel: w950 -> [w959]
                i -> [w964]
                n539 = Increment(x=w964) -> (x+1=w960:i32)
                n540 = Multiply(x=w959, y=w960) -> (x*y=w958:dbl)
                n541 = Add(x=w961, y=w958) -> (x+y=w957:dbl)
                n542 = Replace Array Subset(array=w963, new element=w957, index=w960) -> (w962:dbl[])
              }
            }
            n543 = local read "Concetrations"() -> (w888:dbl[])
            n544 = Divide(x=w893, y=w892) -> (x/y=w890:dbl[][])
            n545 = case shown="False" w889 {
              tunnel: [w915 w927] -> w884
